vi "pixeltolamda.vi"(2 "Grating:":u16(ring) items=["Shimadzu 30-006  "], 3 "Pixel Postion":dbl, 4 "Caibration Date":u16(ring) items=["first calibration - 7/31", "7/31-current"]) -> (0 "E (J)":dbl, 1 "lamda (m)":dbl)   [LabVIEW 2019]
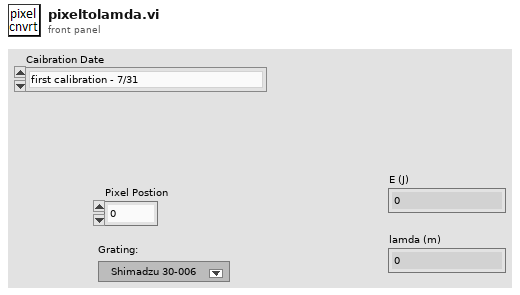
[diagram p1: front panel]
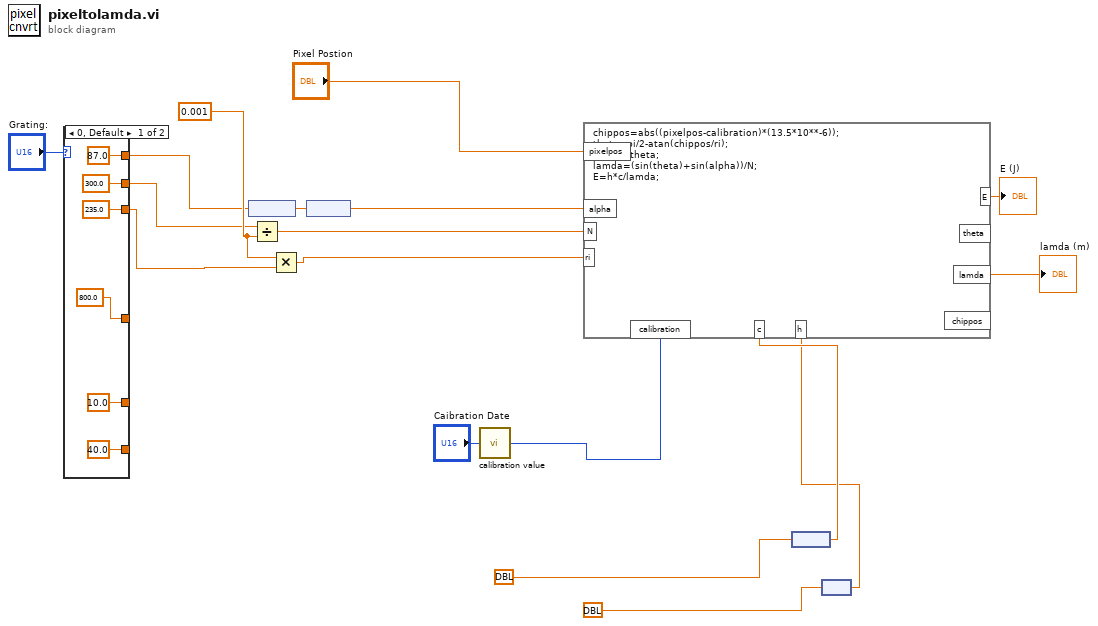
[diagram p0: block diagram]
diagram:
  w16 = 0.001 ("y")
  n1 = case shown="0, Default" "Grating:" {
    tunnel: [300.0 _] -> w14
    tunnel: [87.0 _] -> w15
    tunnel: [10.0 _] -> _
    tunnel: [40.0 _] -> _
    tunnel: [235.0 _] -> w13
    tunnel: [800.0 _] -> _
    frame 0, Default {
    }
    frame 1 {
    }
  }
  n2 = node(w15) -> (w17:dbl[unit])
  n3 = Divide(x=w14, y=w16) -> (x/y=w11:dbl)
  n4 = Multiply(x=w16, y=w13) -> (x*y=w10:dbl)
  n5 = node(w17) -> (w12:dbl)
  n6 = call "calibration value.vi"("Caibration Date"="Caibration Date") -> ("Numeric"=w2:i32)
  n7 = node(ext[unit] 299792458.0) -> (w6:ext)
  n8 = node(ext[unit] 6.62607004e-34) -> (w4:ext)
  n9 = formula code="chippos=abs((pixelpos-calibration)*(13.5*10**-6));\ntheta=pi/2-atan(chippos/ri);\ntheta=-theta;\nlamda=(sin(theta)+sin(alpha))/N;\nE=h*c/lamda;"("N"=w11, "alpha"=w12, "ri"=w10, "pixelpos"="Pixel Postion", "calibration"=w2, "h"=w4, "c"=w6) -> ("lamda"=→"lamda (m)":dbl, "E"=→"E (J)":dbl)  [unwired: 2 out]
